vi "iram_time_frame.vi"() -> ()   [LabVIEW 2017]
uses:
  <vilib>/gmath/NI_Gmath.lvlib
panel:
  out "r 11":dbl format="%.7g"
  out "r 10":dbl format="%.7g"
  out "r 9":dbl format="%.7g"
  out "meannel normált eredõ SNR":cluster{dbl[], dbl[]}(graph)
  out "normált X SNR (szum/time)":cluster{dbl[], dbl[]}(graph)
  out "normált X SNR (imp mean) (0,2Hz 3 felh)":cluster{dbl[], dbl[]}(graph)
  out "r 8":dbl format="%.7g"
  out "r 7":dbl format="%.7g"
  out "r 6":dbl format="%.7g"
  out "r 5":dbl format="%.7g"
  out "r 4":dbl format="%.7g"
  out "r 3":dbl format="%.7g"
  out "r 2":dbl format="%.7g"
  out "r":dbl format="%.7g"
  out "impulse szum/mean":cluster{"X":dbl, "Y":dbl}[](graph)
  in  "felharmonikus N":i32=3
  in  "SNR window width [Hz]":dbl=0.2 format="%#_13g"
  out "impulse mean (egész jó)":cluster{"X":dbl, "Y":dbl}[](graph)
  out "impulse szum":cluster{"X":dbl, "Y":dbl}[](graph)
  out "impulse sd":cluster{"X":dbl, "Y":dbl}[](graph)
  out "impulse szum/time":cluster{"X":dbl, "Y":dbl}[](graph)
  out "X SNR (6min 0,2 Hz, 0 felharmonikus)":cluster{"X":dbl, "Y":dbl}[](graph)
  out "resultant SNR (0,2 Hz 0 felh.)":cluster{"X":dbl, "Y":dbl}[](graph)
  out "X SNR (6min 0,2 Hz, 0 felharmonikus)":cluster{"X":dbl, "Y":dbl}[](graph)
  in  "Path":path=path "C:/Users/Lenovo/Desktop/szakdoga/data/time/egyenletes_resztavok"
  # "ez"
  # "ez"
  # "ez"
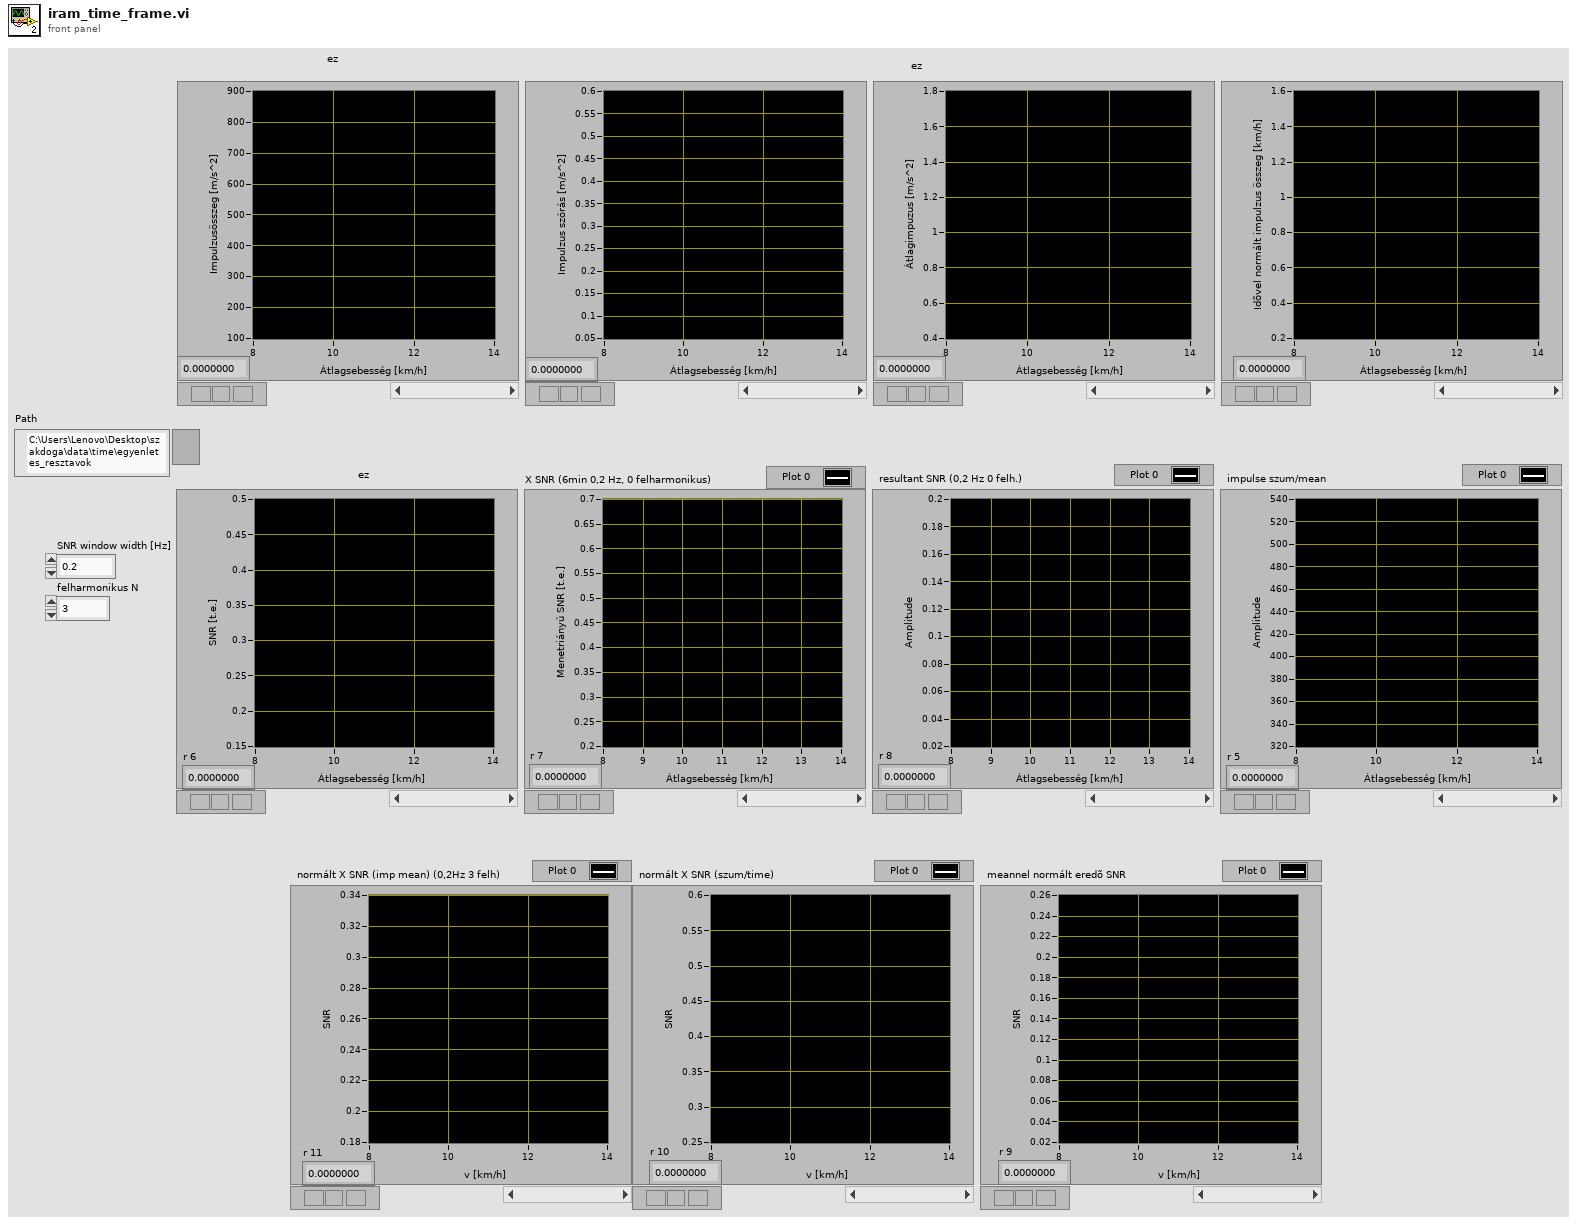
[diagram p1: front panel]
types:
  T1 = cluster{cluster{dbl, "impulse szum/time":dbl}[], cluster{dbl, "impulse  szum":dbl}[], cluster{dbl, "impulse standard deviation":dbl}[], cluster{dbl, "impulse mean":dbl}[], cluster{dbl, "X SNR 1":dbl}[], cluster{dbl, "X SNR 2":dbl}[], cluster{dbl, "X SNR 3":dbl}[], cluster{dbl, "impulse szum/avg":dbl}[]}
  T2 = cluster{cluster{dbl, dbl}[], cluster{dbl, "impulse  szum":dbl}[], cluster{dbl, "impulse standard deviation":dbl}[], cluster{dbl, "impulse mean":dbl}[], cluster{dbl, dbl}[], cluster{dbl, dbl}[], cluster{dbl, dbl}[], cluster{dbl, "impulse szum/mean":dbl}[]}
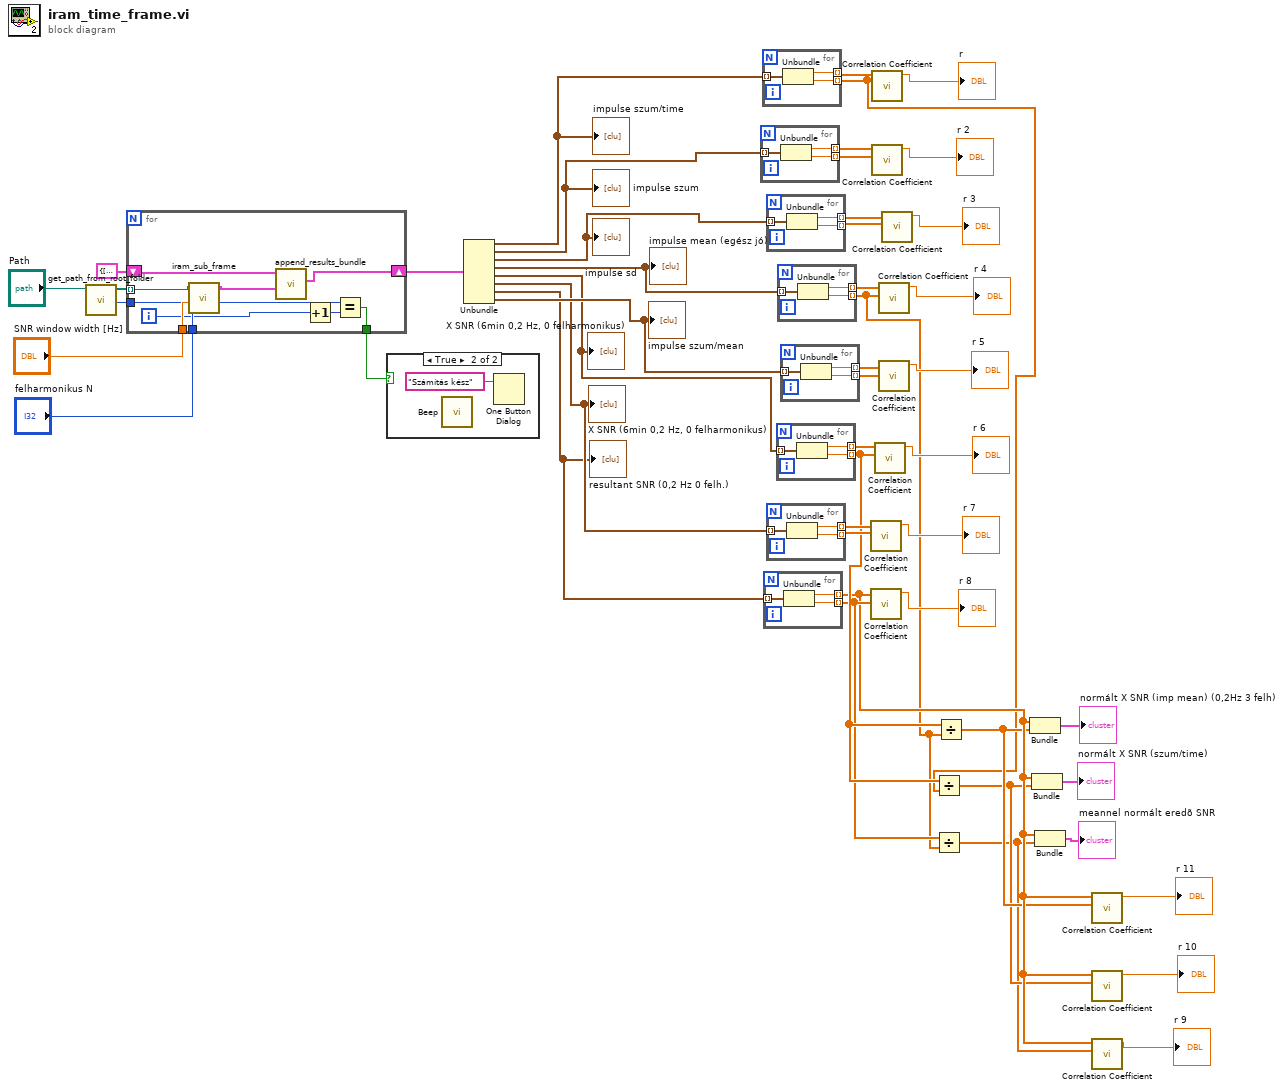
[diagram p0: block diagram]
diagram:
  n1 = call "get_path_from_root_folder.vi"("Path"="Path") -> ("Number of Files"=w45:i32, "Array"=w49:path[])  [unwired: 9 in]
  n2 = for {
    tunnel: w49 -> [w57] mode=indexing
    tunnel: "SNR window width [Hz]" -> [w55]
    tunnel: "felharmonikus N" -> [w54]
    tunnel: w45 -> [w53]
    tunnel: [w50] -> w44
    shift-right: [w58] -> w42
    shift-left: T1 {[], [], [], [], [], [], [], []} ("concat(X,Y)") -> [w59]
    i -> [w51]
    n3 = call "iram_sub_frame.vi"("felharmonikus N"=w54, "SNR window width [Hz]"=w55, "path to binary file"=w57) -> ("output cluster"=w56:T2)  [unwired: 8 in]
    n4 = call "append_results_bundle.vi"("Y"=w56, "X"=w59) -> ("concat(X,Y)"=w58:T1)  [unwired: 8 in]
    n5 = Increment(x=w51) -> (x+1=w52:i32)
    n6 = Equal?(x=w53, y=w52) -> (x = y?=w50:bool)
  }
  n7 = case shown="True" w44 {
    frame False {
    }
    frame True {
      n8 = call <vilib>:"Beep.vi"() -> ()  [unwired: 12 in]
      n9 = One Button Dialog(message="Számítás kész") -> ()  [unwired: 1 in, 1 out]
    }
  }
  n10 = Unbundle(w42) -> (w41:cluster{dbl, "impulse szum/time":dbl}[], w40:cluster{dbl, "impulse  szum":dbl}[], w39:cluster{dbl, "impulse standard deviation":dbl}[], w38:cluster{dbl, "impulse mean":dbl}[], w36:cluster{dbl, "X SNR 1":dbl}[], w35:cluster{dbl, "X SNR 2":dbl}[], w34:cluster{dbl, "X SNR 3":dbl}[], w37:cluster{dbl, "impulse szum/avg":dbl}[])
  "X SNR (6min 0,2 Hz, 0 felharmonikus)" <- w36
  "resultant SNR (0,2 Hz 0 felh.)" <- w34
  "X SNR (6min 0,2 Hz, 0 felharmonikus)" <- w35
  "impulse szum/time" <- w41
  "impulse sd" <- w39
  "impulse szum" <- w40
  "impulse mean (egész jó)" <- w38
  "impulse szum/mean" <- w37
  n11 = for {
    tunnel: w40 -> [w63] mode=indexing
    tunnel: [w62] -> w29 mode=indexing
    tunnel: [w61] -> w13 mode=indexing
    n12 = Unbundle(w63) -> (w62:dbl, "impulse  szum"=w61:dbl)
  }
  n13 = for {
    tunnel: w41 -> [w66] mode=indexing
    tunnel: [w65] -> w33 mode=indexing
    tunnel: [w64] -> w2 mode=indexing
    n14 = Unbundle(w66) -> (w65:dbl, "impulse szum/time"=w64:dbl)
  }
  n15 = for {
    tunnel: w34 -> [w69] mode=indexing
    tunnel: [w68] -> w7 mode=indexing
    tunnel: [w67] -> w11 mode=indexing
    n16 = Unbundle(w69) -> (w68:dbl, "X SNR 3"=w67:dbl)
  }
  n17 = for {
    tunnel: w39 -> [w72] mode=indexing
    tunnel: [w71] -> w21 mode=indexing
    tunnel: [w70] -> w3 mode=indexing
    n18 = Unbundle(w72) -> (w71:dbl, "impulse standard deviation"=w70:dbl)
  }
  n19 = for {
    tunnel: w35 -> [w75] mode=indexing
    tunnel: [w74] -> w18 mode=indexing
    tunnel: [w73] -> w17 mode=indexing
    n20 = Unbundle(w75) -> (w74:dbl, "X SNR 2"=w73:dbl)
  }
  n21 = for {
    tunnel: w36 -> [w78] mode=indexing
    tunnel: [w77] -> w19 mode=indexing
    tunnel: [w76] -> w12 mode=indexing
    n22 = Unbundle(w78) -> (w77:dbl, "X SNR 1"=w76:dbl)
  }
  n23 = for {
    tunnel: w38 -> [w81] mode=indexing
    tunnel: [w80] -> w31 mode=indexing
    tunnel: [w79] -> w1 mode=indexing
    n24 = Unbundle(w81) -> (w80:dbl, "impulse mean"=w79:dbl)
  }
  n25 = for {
    tunnel: w37 -> [w84] mode=indexing
    tunnel: [w83] -> w30 mode=indexing
    tunnel: [w82] -> w20 mode=indexing
    n26 = Unbundle(w84) -> (w83:dbl, "impulse szum/avg"=w82:dbl)
  }
  n27 = call <vilib>:"Correlation Coefficient.vi"("Y"=w17, "X"=w18) -> ("correlation coefficient r"=→"r 7":dbl)  [unwired: 8 in, 1 out]
  n28 = call <vilib>:"Correlation Coefficient.vi"("Y"=w11, "X"=w7) -> ("correlation coefficient r"=→"r 8":dbl)  [unwired: 8 in, 1 out]
  n29 = call <vilib>:"Correlation Coefficient.vi"("Y"=w2, "X"=w33) -> ("correlation coefficient r"=→"r":dbl)  [unwired: 8 in, 1 out]
  n30 = call <vilib>:"Correlation Coefficient.vi"("Y"=w13, "X"=w29) -> ("correlation coefficient r"=→"r 2":dbl)  [unwired: 8 in, 1 out]
  n31 = call <vilib>:"Correlation Coefficient.vi"("Y"=w12, "X"=w19) -> ("correlation coefficient r"=→"r 6":dbl)  [unwired: 8 in, 1 out]
  n32 = call <vilib>:"Correlation Coefficient.vi"("Y"=w1, "X"=w31) -> ("correlation coefficient r"=→"r 4":dbl)  [unwired: 8 in, 1 out]
  n33 = call <vilib>:"Correlation Coefficient.vi"("Y"=w20, "X"=w30) -> ("correlation coefficient r"=→"r 5":dbl)  [unwired: 8 in, 1 out]
  n34 = call <vilib>:"Correlation Coefficient.vi"("Y"=w3, "X"=w21) -> ("correlation coefficient r"=→"r 3":dbl)  [unwired: 8 in, 1 out]
  n35 = Divide(x=w12, y=w2) -> (x/y=w5:dbl[])
  n36 = Divide(x=w11, y=w1) -> (x/y=w4:dbl[])
  n37 = Divide(x=w12, y=w1) -> (x/y=w6:dbl[])
  n38 = Bundle(w7, w6) -> (→"normált X SNR (imp mean) (0,2Hz 3 felh)":cluster{dbl[], dbl[]})  [unwired: 1 in]
  n39 = Bundle(w7, w5) -> (→"normált X SNR (szum/time)":cluster{dbl[], dbl[]})  [unwired: 1 in]
  n40 = Bundle(w7, w4) -> (→"meannel normált eredõ SNR":cluster{dbl[], dbl[]})  [unwired: 1 in]
  n41 = call <vilib>:"Correlation Coefficient.vi"("Y"=w6, "X"=w7) -> ("correlation coefficient r"=→"r 11":dbl)  [unwired: 8 in, 1 out]
  n42 = call <vilib>:"Correlation Coefficient.vi"("Y"=w5, "X"=w7) -> ("correlation coefficient r"=→"r 10":dbl)  [unwired: 8 in, 1 out]
  n43 = call <vilib>:"Correlation Coefficient.vi"("Y"=w4, "X"=w7) -> ("correlation coefficient r"=→"r 9":dbl)  [unwired: 8 in, 1 out]
